vi "Write Port.vi"(8 "error in":errorcluster, 10 "port":u16, 11 "TCP slave in":refnum<class "TCP Server.lvclass">) -> (0 "error out":errorcluster, 3 "TCP slave out":refnum<class "TCP Server.lvclass">)   [LabVIEW 2021, in "WebSockets.lvlib" / "TCP Server.lvclass"]
doc: "Property accessor for the TCP port."
uses:
  TCP Server.lvclass
  C:/my_projects/projects/Algorithms/Labview/21/WebSockets/Source/WebSockets/WebSocket/WebSocket.lvclass
  WebSocket/WebSocket.lvclass/WebSocket.ctl
  Sockets/VISA TCP Socket/VISA TCP.lvclass
  C:/my_projects/projects/Algorithms/Labview/21/WebSockets/Source/Sockets/Socket/Socket.lvclass
  Sockets/VISA TCP Socket/VISA TCP.lvclass/VISA TCP.ctl
  WebSocket/WebSocket.lvclass
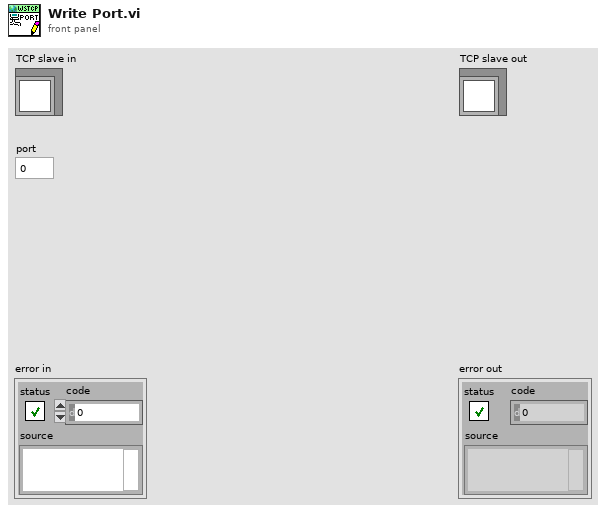
[diagram p1: front panel]
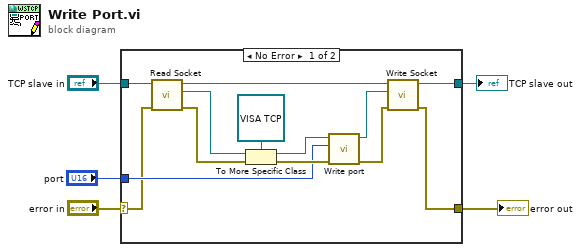
[diagram p0: block diagram]
diagram:
  n1 = case shown="No Error" "error in" {
    selector: "error in" -> [w6 w20]
    tunnel: "TCP slave in" -> [w15 w19]
    tunnel: "port" -> [w12 _]
    tunnel: [w8 w20] -> w3
    tunnel: [w7 w19] -> w2
    frame No Error {
      n2 = call "Read Socket.vi"("error in (no error)"=w6, "WebSocket in"=w15) -> ("error out"=w16:errorcluster, "Socket"=w17:refnum<class "Socket.lvclass">, "WebSocket out"=w10:refnum<class "TCP Server.lvclass">)  [unwired: 7 in]
      n3 = To More Specific Class(target class=refnum<class "VISA TCP.lvclass"> refnum ("Sockets:VISA TCP"), reference=w17, error in=w16) -> (specific class reference=w13:refnum<class "VISA TCP.lvclass">, error out=w14:errorcluster)
      n4 = call "Write port.vi"("error in (no error)"=w14, "port"=w12, "VISA TCP in"=w13) -> ("error out"=w9:errorcluster, "VISA TCP out"=w11:refnum<class "VISA TCP.lvclass">)  [unwired: 7 in]
      n5 = call "Write Socket.vi"("error in (no error)"=w9, "Socket"=w11, "WebSocket in"=w10) -> ("error out"=w8:errorcluster, "WebSocket out"=w7:refnum<class "TCP Server.lvclass">)  [unwired: 7 in]
    }
    frame Error {
    }
  }
  "error out" <- w3
  "TCP slave out" <- w2
